vi "Measurement Functional Variable_Meas-Scope SP.vi"(1 "Mode(Get)":T2=enum."Get", 7 "MeasuConfig":T1={"Para."={"Chans"=[], "LevelRange"={"Max"=10.0, "Min"=-10.0}, "InstruHandle"=""}, "Value"=[]}) -> (8 "MeasuConfig":T1={"Para."={"Chans"=[], "LevelRange"={"Max"=10.0, "Min"=-10.0}, "InstruHandle"=""}, "Value"=[]})   [LabVIEW 2012]
doc: "功能全局，用于保存程序运行中添加的测量量。"
uses:
  Data Structure.llb/Function Variable Parameter Operations-Scope SP.ctl
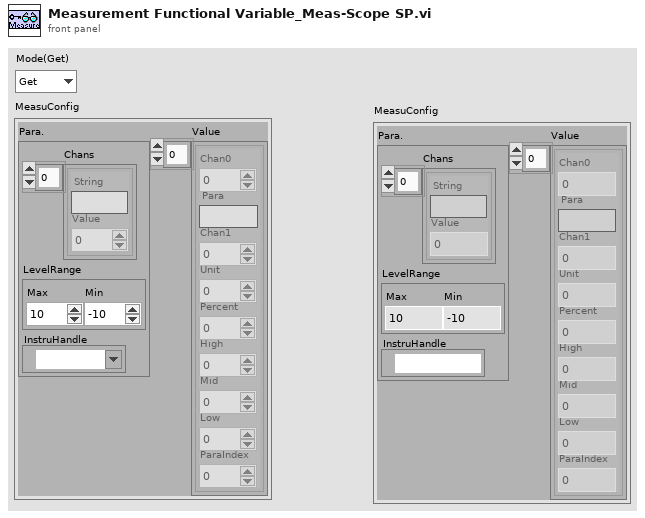
[diagram p1: front panel]
types:
  T1 = cluster{"Para.":cluster{"Chans":cluster{"String":string, "Value":ext}[], "LevelRange":cluster{"Max":dbl, "Min":dbl}, "InstruHandle":refnum<k15>}, "Value":cluster{"Chan0":i32, "Para":string, "Chan1":i32, "Unit":i32, "Percent":i32, "High":dbl, "Mid":dbl, "Low":dbl, "ParaIndex":i32}[]}
  T2 = typedef "Function Variable Parameter Operations-Scope SP.ctl" = enum16{"Set", "Get"}
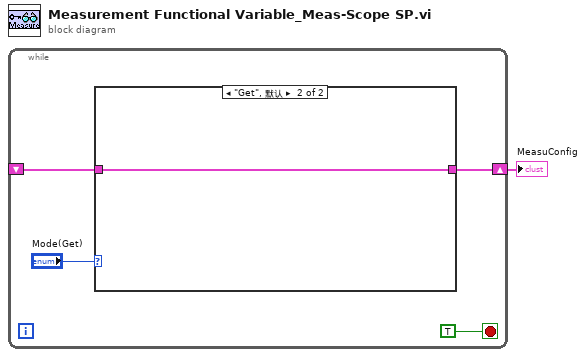
[diagram p0: block diagram]
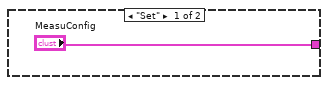
[diagram p2: hidden frame]
diagram:
  n1 = while {
    shift-right: [w5] -> w1
    shift-left: _ -> [w3]
    stop <- TRUE stop-if-true
    n2 = case shown="\"Get\", 默认" "Mode(Get)" {
      tunnel: ["MeasuConfig" w7] -> w5
      tunnel: w3 -> [_ w7]
      frame "Set" {
      }
      frame "Get", Default {
      }
    }
  }
  "MeasuConfig" <- w1
